vi "Calibrate AI Raw.vi"(1 "Calibration Data":T1[](array[typedef]), 2 "AI Raw":sgl[](array[numeric])=[0.0, 0.0, 0.0, 0.0]) -> (5 "AI Calibrated":sgl[](array[numeric]))   [LabVIEW 2020]
uses:
  Control/Cluster - Calibration Data.ctl
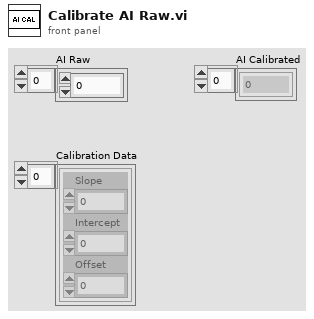
[diagram p1: front panel]
types:
  T1 = typedef "Cluster - Calibration Data.ctl" = cluster{"Slope":sgl, "Intercept":sgl, "Offset":sgl}
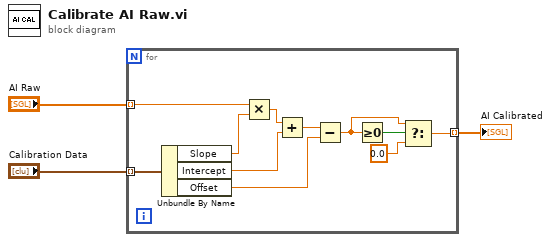
[diagram p0: block diagram]
diagram:
  n1 = for {
    tunnel: "AI Raw" -> [w13] mode=indexing
    tunnel: "Calibration Data" -> [w14] mode=indexing
    tunnel: [w4] -> w3 mode=indexing
    n2 = Unbundle By Name(w14) -> ("Slope"=w12:sgl, "Intercept"=w10:sgl, "Offset"=w8:sgl)
    n3 = Multiply(x=w13, y=w12) -> (x*y=w11:sgl)
    n4 = Add(x=w11, y=w10) -> (x+y=w9:sgl)
    n5 = Subtract(x=w9, y=w8) -> (x-y=w6:sgl)
    n6 = Greater Or Equal To 0?(x=w6) -> (x >= 0?=w7:bool)
    n7 = Select(t=w6, s=w7, f=sgl 0.0) -> (s? t:f=w4:sgl)
  }
  "AI Calibrated" <- w3
